vi "setting page 2.vi"() -> (15 "This VI":refnum<vi>)   [LabVIEW 2019]
uses:
  database.lvlib
panel:
  in  "counting device":enum16{"Sensors", "Line Speed", "Sensors&Speed"}(ring)
  in  "IP # speed":string="169.254.12.252"
  out "Error out 7":errorcluster
  out "Error out 6":errorcluster
  out "Error out 5":errorcluster
  out "Error out 4":errorcluster
  out "Error out 3":errorcluster
  out "Error out 2":errorcluster
  out "Error out":errorcluster
  in  "Close Square":bool
  in  "madule path":path=path "C:/Users/DPIS/Desktop/dpis2022/Pallet-car-master/Pallet-car-master/main_func.py"
  in  "high level read thr 3":dbl=25000.0
  in  "high level read thr 2":dbl=25000.0
  in  "box ratio":dbl=8.0
  out "error constant 2":errorcluster
  in  "DB days to save":i16=3
  in  "Debounce Time (s)":dbl=1.0
  in  "counting role 2":T1(ring) caption="counting role"
  in  "ch sw sensor1":dbl
  out "Side Wall Setting":string
  in  "Port":u16=502
  in  "SWL thr":dbl=5000.0
  in  "high level read thr 1":dbl=25000.0
  in  "rising level thr":dbl=50.0
  in  "Database Name":string="dsgs"
  in  "plt number dis":i16=45
  in  "Table Name":string="dpis"
  out "General Setting":string
  in  "SW timout(s)":dbl=1.0
  in  "Curv thr (mm)":dbl=13.0
  in  "SWR thr":dbl=5000.0
  in  "ch sw sensor2":dbl=1.0
  in  "ch sensor3":dbl=6.0
  in  "ch sensor2":dbl=4.0
  in  "ch sensor1":dbl=2.0
  in  "falling Thr sensor 3":dbl=20000.0
  out "Gratebar Setting":string
  in  "max area (hole)":dbl=6000.0
  in  "min area (hole)":dbl=2000.0
  in  "max area size (gap)":dbl=2000.0
  in  "min area size(gap)":dbl=550.0
  in  "max box size":dbl=300000.0
  in  "min box size":dbl=100000.0
  in  "IP #":string="169.254.50.68"
  out "Curve Setting":string
  in  "Img Path":path=path "C:/Users/DPIS/Pictures/pallet pics"
  in  "level2 thr %":u16=50
  in  "level1 thr %":u16=26
  in  "time out":u16=50
  in  "falling Thr sensor 2":dbl=20000.0
  in  "falling Thr sensor 1":dbl=20000.0
  # "DPIS"
  # "SETTING"
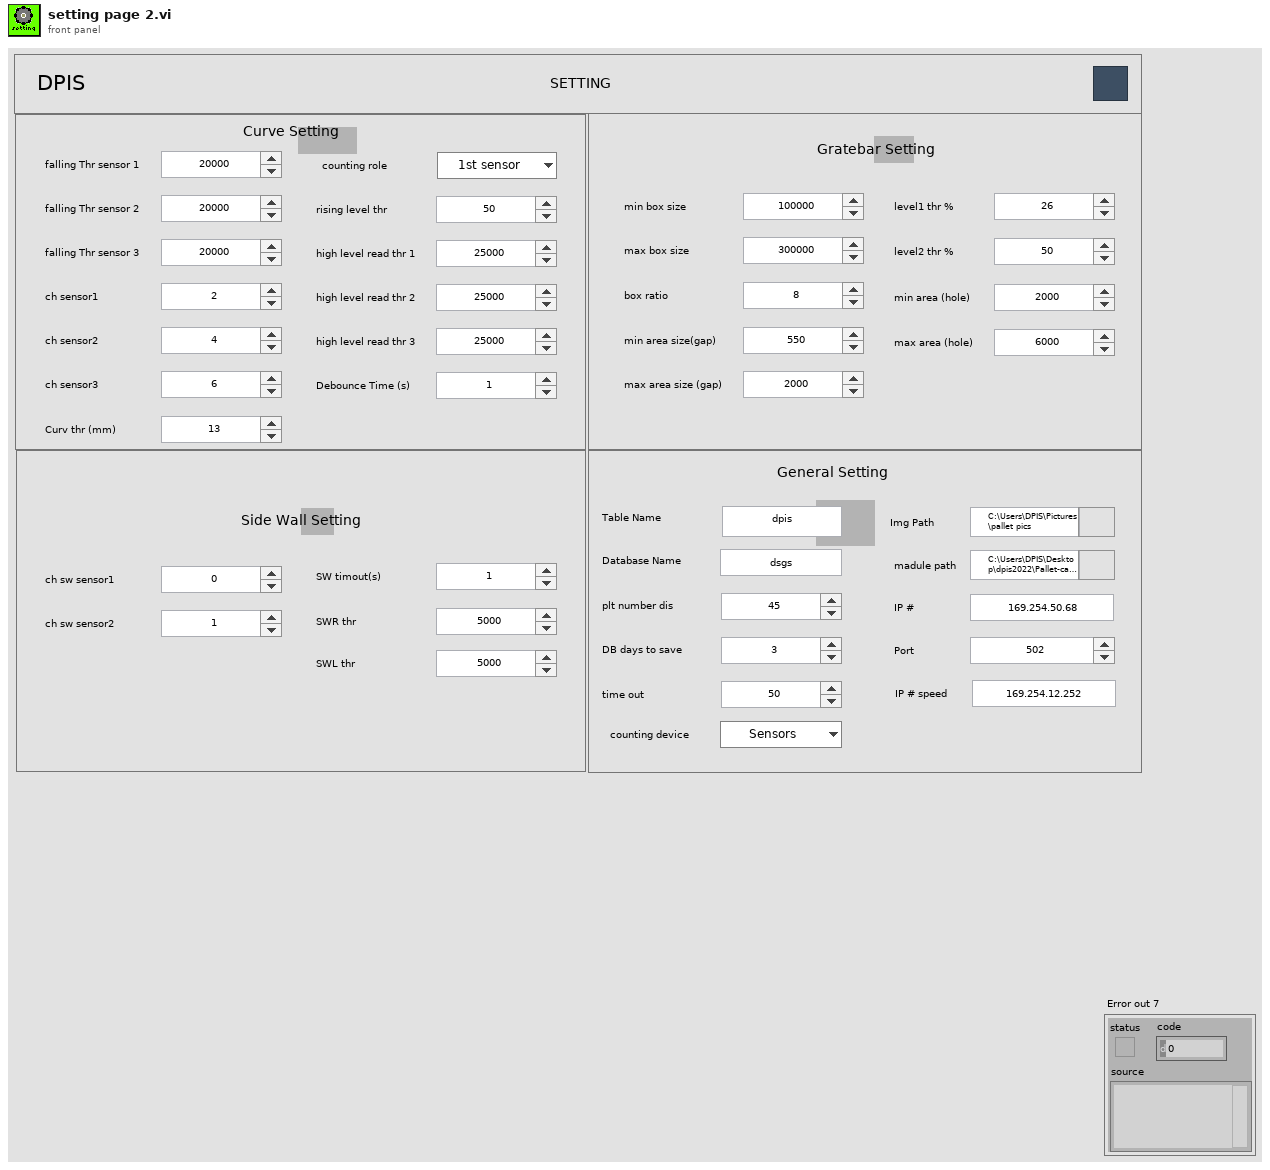
[diagram p1: front panel]
types:
  T1 = enum16{"1st sensor", "2nd sensor", "3rd sensor", "1st+2nd", "1st+3rd", "2nd+3rd", "1st+2nd+3rd"}
  T2 = cluster{i32, string, string, i32, string, path, i32, i32, path, string, "Value":enum16{"Sensors", "Line Speed", "Sensors&Speed"}}
  T3 = cluster{"min box size":dbl, "max box size":dbl, "box ratio":dbl, "min area size(gap)":dbl, "max area size (gap)":dbl, "min area (hole)":dbl, "max area (hole)":dbl}
  T4 = cluster{"ch sensor1":dbl, "ch sensor2":dbl, "chs ensor3":dbl, "ch sw sensor1":dbl, "ch sw sensor2":dbl}
  T5 = cluster{"plt number dis":i16, "Table Name":string, "Database Name":string, "DB days to save":i16, "IP #":string, "Img Path":path, "Port":u16, "time out":u16, "madule path":path}
  T6 = cluster{"high level read thr 1":dbl, "high level read thr 2":dbl, "high level read thr 3":dbl, "Debounce Time (s)":dbl, "rising level thr":dbl, "counting role 2":enum16{"1st sensor", "2nd sensor", "3rd sensor", "1st+2nd", "1st+3rd", "2nd+3rd", "1st+2nd+3rd"}}
  T7 = cluster{"Curv thr (mm)":dbl, "SW timout(s)":dbl, "SWR thr":dbl, "SWL thr ":dbl}
  T8 = cluster{"plt number dis":i16, "Table Name":string, "Database Name":string, "DB days to save":i16, "IP #":string, "Img Path":path, "Port":u16, "time out":u16, "madule path":path, "IP # speed":string, "counting device":enum16{"Sensors", "Line Speed", "Sensors&Speed"}}
  T9 = cluster{"falling Thr sensor 1":dbl, "falling Thr sensor 2":dbl, "falling Thr sensor 3":dbl}
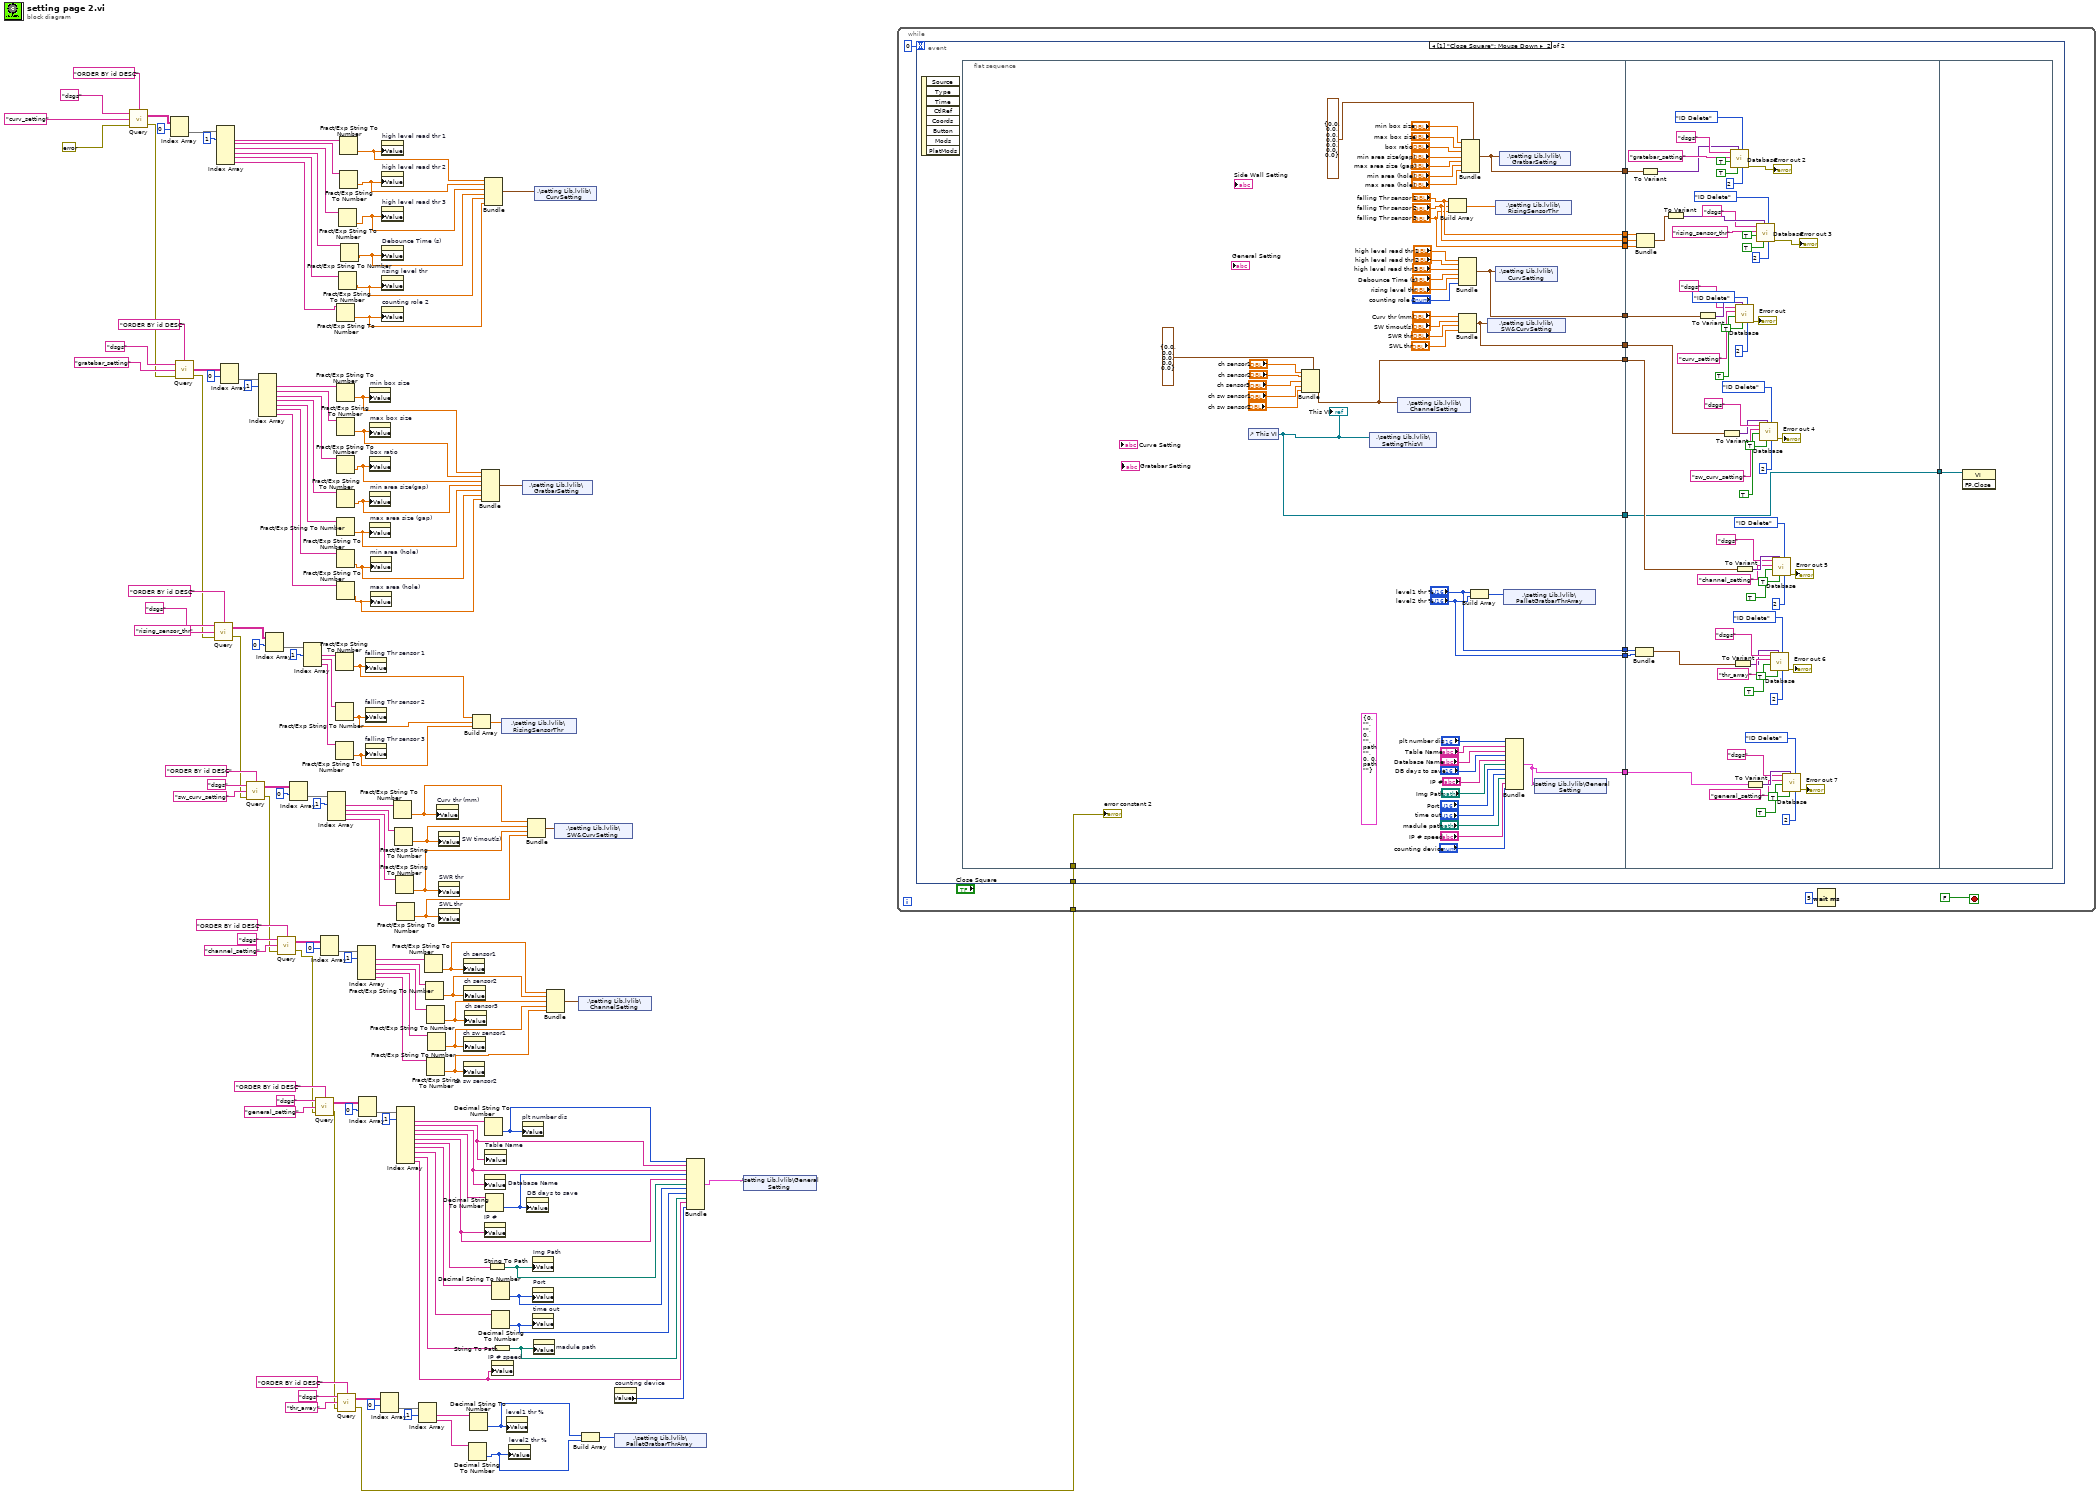
[diagram p0: block diagram]
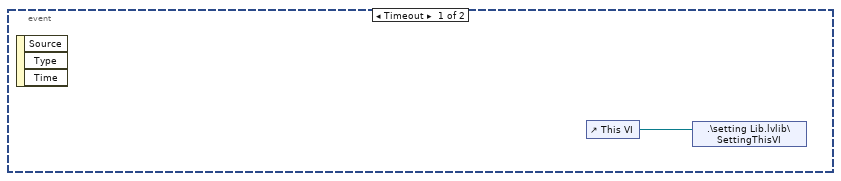
[diagram p2: hidden frame]
diagram:
  n1 = call "Query.vi"("Condition"="ORDER BY id DESC", "Error in"=errorcluster {"status"=FALSE, "code"=0, "source"=""}, "Table Name"="curv_setting", "Connection Name"="dsgs") -> ("Error out"=w106:errorcluster, "data"=w129:string[][])
  n2 = Index Array(array=w129, index (row)=0) -> (element=w131:string[])  [unwired: 1 in]
  n3 = call "Query.vi"("Condition"="ORDER BY id DESC", "Error in"=w106, "Table Name"="gratebar_setting", "Connection Name"="dsgs") -> ("Error out"=w83:errorcluster, "data"=w112:string[][])
  n4 = call "Query.vi"("Condition"="ORDER BY id DESC", "Error in"=w83, "Table Name"="rising_sensor_thr", "Connection Name"="dsgs") -> ("Error out"=w68:errorcluster, "data"=w85:string[][])
  n5 = Index Array(array=w131, index #1=1 ("index")) -> (element #1=w125:string, element #2=w124:string, element #3=w123:string, element #4=w126:string, element #5=w122:string, element #6=w121:string)  [unwired: 5 in]
  n6 = Index Array(array=w112, index (row)=0) -> (element=w110:string[])  [unwired: 1 in]
  n7 = call "Query.vi"("Condition"="ORDER BY id DESC", "Error in"=w68, "Table Name"="sw_curv_setting", "Connection Name"="dsgs") -> ("Error out"=w47:errorcluster, "data"=w74:string[][])
  n8 = Index Array(array=w110, index #1=1 ("index")) -> (element #1=w105:string, element #2=w104:string, element #3=w103:string, element #4=w102:string, element #5=w101:string, element #6=w100:string, element #7=w99:string)  [unwired: 6 in]
  n9 = Index Array(array=w85, index (row)=0) -> (element=w87:string[])  [unwired: 1 in]
  n10 = call "Query.vi"("Condition"="ORDER BY id DESC", "Error in"=w47, "Table Name"="channel_setting", "Connection Name"="dsgs") -> ("Error out"=w32:errorcluster, "data"=w49:string[][])
  n11 = Index Array(array=w74, index (row)=0) -> (element=w72:string[])  [unwired: 1 in]
  n12 = Index Array(array=w87, index #1=1 ("index")) -> (element #1=w82:string, element #2=w81:string, element #3=w80:string)  [unwired: 2 in]
  n13 = call "Query.vi"("Condition"="ORDER BY id DESC", "Error in"=w32, "Table Name"="general_setting", "Connection Name"="dsgs") -> ("Error out"=w9:errorcluster, "data"=w38:string[][])
  n14 = Index Array(array=w49, index (row)=0) -> (element=w51:string[])  [unwired: 1 in]
  n15 = Index Array(array=w72, index #1=1 ("index")) -> (element #1=w67:string, element #2=w66:string, element #3=w65:string, element #4=w64:string)  [unwired: 3 in]
  n16 = Fract/Exp String To Number(string=w82) -> (number=w79:dbl)  [unwired: 3 in, 1 out]
  n17 = Fract/Exp String To Number(string=w81) -> (number=w78:dbl)  [unwired: 3 in, 1 out]
  n18 = Fract/Exp String To Number(string=w80) -> (number=w77:dbl)  [unwired: 3 in, 1 out]
  n19 = Fract/Exp String To Number(string=w105) -> (number=w98:dbl)  [unwired: 3 in, 1 out]
  n20 = Fract/Exp String To Number(string=w104) -> (number=w97:dbl)  [unwired: 3 in, 1 out]
  n21 = Fract/Exp String To Number(string=w103) -> (number=w96:dbl)  [unwired: 3 in, 1 out]
  n22 = Fract/Exp String To Number(string=w102) -> (number=w95:dbl)  [unwired: 3 in, 1 out]
  n23 = Fract/Exp String To Number(string=w101) -> (number=w94:dbl)  [unwired: 3 in, 1 out]
  n24 = Fract/Exp String To Number(string=w121) -> (number=w115:dbl)  [unwired: 3 in, 1 out]
  n25 = Fract/Exp String To Number(string=w100) -> (number=w93:dbl)  [unwired: 3 in, 1 out]
  n26 = Fract/Exp String To Number(string=w99) -> (number=w92:dbl)  [unwired: 3 in, 1 out]
  n27 = call "Query.vi"("Condition"="ORDER BY id DESC", "Error in"=w9, "Table Name"="thr_array", "Connection Name"="dsgs") -> ("Error out"=w135:errorcluster, "data"=w11:string[][])
  n28 = Fract/Exp String To Number(string=w122) -> (number=w116:dbl)  [unwired: 3 in, 1 out]
  n29 = Fract/Exp String To Number(string=w123) -> (number=w118:dbl)  [unwired: 3 in, 1 out]
  n30 = Fract/Exp String To Number(string=w125) -> (number=w120:dbl)  [unwired: 3 in, 1 out]
  n31 = Fract/Exp String To Number(string=w124) -> (number=w119:dbl)  [unwired: 3 in, 1 out]
  n32 = Fract/Exp String To Number(string=w126) -> (number=w117:dbl)  [unwired: 3 in, 1 out]
  n33 = Index Array(array=w51, index #1=1 ("index")) -> (element #1=w55:string, element #2=w56:string, element #3=w57:string, element #4=w58:string, element #5=w46:string)  [unwired: 4 in]
  n34 = Index Array(array=w38, index (row)=0) -> (element=w36:string[])  [unwired: 1 in]
  n35 = property on="falling Thr sensor 1" class="DigNum (strict)"("Value"=w79) -> ()  [unwired: 2 in, 2 out]
  n36 = property on="falling Thr sensor 2" class="DigNum (strict)"("Value"=w78) -> ()  [unwired: 2 in, 2 out]
  n37 = property on="falling Thr sensor 3" class="DigNum (strict)"("Value"=w77) -> ()  [unwired: 2 in, 2 out]
  n38 = property on="min box size" class="DigNum (strict)"("Value"=w98) -> ()  [unwired: 2 in, 2 out]
  n39 = property on="max box size" class="DigNum (strict)"("Value"=w97) -> ()  [unwired: 2 in, 2 out]
  n40 = property on="box ratio" class="DigNum (strict)"("Value"=w96) -> ()  [unwired: 2 in, 2 out]
  n41 = property on="min area size(gap)" class="DigNum (strict)"("Value"=w95) -> ()  [unwired: 2 in, 2 out]
  n42 = property on="max area size (gap)" class="DigNum (strict)"("Value"=w94) -> ()  [unwired: 2 in, 2 out]
  n43 = property on="min area (hole)" class="DigNum (strict)"("Value"=w93) -> ()  [unwired: 2 in, 2 out]
  n44 = property on="max area (hole)" class="DigNum (strict)"("Value"=w92) -> ()  [unwired: 2 in, 2 out]
  n45 = Index Array(array=w11, index (row)=0) -> (element=w13:string[])  [unwired: 1 in]
  n46 = property on="high level read thr 1" class="DigNum (strict)"("Value"=w120) -> ()  [unwired: 2 in, 2 out]
  n47 = property on="high level read thr 2" class="DigNum (strict)"("Value"=w119) -> ()  [unwired: 2 in, 2 out]
  n48 = property on="high level read thr 3" class="DigNum (strict)"("Value"=w118) -> ()  [unwired: 2 in, 2 out]
  n49 = property on="Debounce Time (s)" class="DigNum (strict)"("Value"=w117) -> ()  [unwired: 2 in, 2 out]
  n50 = property on="rising level thr" class="DigNum (strict)"("Value"=w116) -> ()  [unwired: 2 in, 2 out]
  n51 = property on="counting role 2" class="Enum (strict)"("Value"=w115) -> ()  [unwired: 2 in, 2 out]
  n52 = Fract/Exp String To Number(string=w67) -> (number=w63:dbl)  [unwired: 3 in, 1 out]
  n53 = Fract/Exp String To Number(string=w66) -> (number=w62:dbl)  [unwired: 3 in, 1 out]
  n54 = Fract/Exp String To Number(string=w65) -> (number=w61:dbl)  [unwired: 3 in, 1 out]
  n55 = Index Array(array=w36, index #1=1 ("index")) -> (element #1=w31:string, element #2=w25:string, element #3=w24:string, element #4=w23:string, element #5=w22:string, element #6=w30:string, element #7=w29:string, element #8=w28:string, element #9=w27:string, element #10=w3:string)  [unwired: 9 in]
  n56 = Fract/Exp String To Number(string=w64) -> (number=w60:dbl)  [unwired: 3 in, 1 out]
  n57 = Index Array(array=w13, index #1=1 ("index")) -> (element #1=w8:string, element #2=w7:string)  [unwired: 1 in]
  n58 = Fract/Exp String To Number(string=w55) -> (number=w45:dbl)  [unwired: 3 in, 1 out]
  n59 = Fract/Exp String To Number(string=w56) -> (number=w44:dbl)  [unwired: 3 in, 1 out]
  n60 = Fract/Exp String To Number(string=w57) -> (number=w43:dbl)  [unwired: 3 in, 1 out]
  n61 = Fract/Exp String To Number(string=w46) -> (number=w41:dbl)  [unwired: 3 in, 1 out]
  n62 = Fract/Exp String To Number(string=w58) -> (number=w42:dbl)  [unwired: 3 in, 1 out]
  n63 = property on="Curv thr (mm)" class="DigNum (strict)"("Value"=w63) -> ()  [unwired: 2 in, 2 out]
  n64 = property on="SW timout(s)" class="DigNum (strict)"("Value"=w62) -> ()  [unwired: 2 in, 2 out]
  n65 = property on="SWR thr" class="DigNum (strict)"("Value"=w61) -> ()  [unwired: 2 in, 2 out]
  n66 = property on="SWL thr" class="DigNum (strict)"("Value"=w60) -> ()  [unwired: 2 in, 2 out]
  n67 = property on="ch sensor1" class="DigNum (strict)"("Value"=w45) -> ()  [unwired: 2 in, 2 out]
  n68 = property on="ch sw sensor2" class="DigNum (strict)"("Value"=w41) -> ()  [unwired: 2 in, 2 out]
  n69 = property on="ch sensor2" class="DigNum (strict)"("Value"=w44) -> ()  [unwired: 2 in, 2 out]
  n70 = property on="ch sw sensor1" class="DigNum (strict)"("Value"=w42) -> ()  [unwired: 2 in, 2 out]
  n71 = property on="ch sensor3" class="DigNum (strict)"("Value"=w43) -> ()  [unwired: 2 in, 2 out]
  n72 = Decimal String To Number(string=w7) -> (number=w4:i32)  [unwired: 2 in, 1 out]
  n73 = Decimal String To Number(string=w8) -> (number=w5:i32)  [unwired: 2 in, 1 out]
  n74 = Build Array(w79, w78, w77) -> (w76:dbl[])
  n75 = Bundle(w98, w97, w96, w95, w94, w93, w92) -> (w91:cluster{dbl, dbl, dbl, dbl, dbl, dbl, dbl})  [unwired: 1 in]
  n76 = Decimal String To Number(string=w31) -> (number=w26:i32)  [unwired: 2 in, 1 out]
  n77 = property on="Database Name" class="Str"("Value"=w24) -> ()  [unwired: 2 in, 2 out]
  n78 = property on="IP #" class="Str"("Value"=w22) -> ()  [unwired: 2 in, 2 out]
  n79 = Bundle(w120, w119, w118, w117, w116, w115) -> (w114:cluster{dbl, dbl, dbl, dbl, dbl, dbl})  [unwired: 1 in]
  n80 = property on="Table Name" class="Str"("Value"=w25) -> ()  [unwired: 2 in, 2 out]
  n81 = Decimal String To Number(string=w23) -> (number=w21:i32)  [unwired: 2 in, 1 out]
  n82 = String To Path(string=w30) -> (path=w20:path)
  n83 = Decimal String To Number(string=w29) -> (number=w19:i32)  [unwired: 2 in, 1 out]
  n84 = Decimal String To Number(string=w28) -> (number=w18:i32)  [unwired: 2 in, 1 out]
  n85 = property on="IP # speed" class="Str"("Value"=w3) -> ()  [unwired: 2 in, 2 out]
  n86 = String To Path(string=w27) -> (path=w17:path)
  n87 = shared-variable ".\\setting Lib.lvlib\\RisingSensorThr"(w76) -> ()  [unwired: 1 in, 1 out]
  n88 = property on="level1 thr %" class="DigNum (strict)"("Value"=w5) -> ()  [unwired: 2 in, 2 out]
  n89 = property on="level2 thr %" class="DigNum (strict)"("Value"=w4) -> ()  [unwired: 2 in, 2 out]
  n90 = shared-variable ".\\setting Lib.lvlib\\GratbarSetting"(w91) -> ()  [unwired: 1 in, 1 out]
  n91 = property on="plt number dis" class="DigNum (strict)"("Value"=w26) -> ()  [unwired: 2 in, 2 out]
  n92 = property on="DB days to save" class="DigNum (strict)"("Value"=w21) -> ()  [unwired: 2 in, 2 out]
  n93 = Bundle(w63, w62, w61, w60) -> (w59:cluster{dbl, dbl, dbl, dbl})  [unwired: 1 in]
  n94 = property on="Img Path" class="Path"("Value"=w20) -> ()  [unwired: 2 in, 2 out]
  n95 = property on="Port" class="DigNum (strict)"("Value"=w19) -> ()  [unwired: 2 in, 2 out]
  n96 = property on="time out" class="DigNum (strict)"("Value"=w18) -> ()  [unwired: 2 in, 2 out]
  n97 = property on="madule path" class="Path"("Value"=w17) -> ()  [unwired: 2 in, 2 out]
  n98 = shared-variable ".\\setting Lib.lvlib\\CurvSetting"(w114) -> ()  [unwired: 1 in, 1 out]
  n99 = Bundle(w45, w44, w43, w42, w41) -> (w40:cluster{dbl, dbl, dbl, dbl, dbl})  [unwired: 1 in]
  n100 = shared-variable ".\\setting Lib.lvlib\\SW&CurvSetting"(w59) -> ()  [unwired: 1 in, 1 out]
  n101 = shared-variable ".\\setting Lib.lvlib\\ChannelSetting"(w40) -> ()  [unwired: 1 in, 1 out]
  n102 = Build Array(w5, w4) -> (w6:i32[])
  n103 = shared-variable ".\\setting Lib.lvlib\\PalletGratbarThrArray"(w6) -> ()  [unwired: 1 in, 1 out]
  n104 = property on="counting device" class="Enum (strict)"() -> ("Value"=w1:enum16{"Sensors", "Line Speed", "Sensors&Speed"})  [unwired: 2 in, 2 out]
  n105 = Bundle(w26, w25, w24, w21, w22, w20, w19, w18, w17, w3, "Value"=w1) -> (w2:T2)  [unwired: 1 in]
  n106 = shared-variable ".\\setting Lib.lvlib\\General Setting"(w2) -> ()  [unwired: 1 in, 1 out]
  n107 = while {
    tunnel: w135 -> [w138]
    stop <- FALSE stop-if-true
    n108 = event shown="[1] \"Close Square\": Mouse Down" {
      selector: _ -> [_ _]
      dyn-events: _ -> [_ _]
      timeout: 0 -> [_ _]
      tunnel: w138 -> [_ w143]
      event Timeout {
        n109 = event-data() -> ()  [unwired: 1 in, 3 out]
        n110 = control-ref of="This VI"() -> (w140:refnum<vi>)
        n111 = shared-variable ".\\setting Lib.lvlib\\SettingThisVI"(w140) -> ()  [unwired: 1 in, 1 out]
      }
      event "Close Square": Mouse Down {
        n112 = event-data() -> ()  [unwired: 1 in, 8 out]
        n113 = flat-sequence {
          tunnel: ["falling Thr sensor 1"] -> w153
          tunnel: ["falling Thr sensor 2"] -> w152
          tunnel: ["falling Thr sensor 3"] -> w151
          tunnel: [w165] -> w150
          tunnel: [w164] -> w149
          tunnel: [w163] -> w148
          tunnel: [w161] -> w147
          tunnel: ["level1 thr %"] -> w146
          tunnel: ["level2 thr %"] -> w145
          tunnel: [w154] -> w144
          tunnel: w143 -> [w158]
          tunnel: [w157] -> w141
          tunnel: w153 -> [w248]
          tunnel: w152 -> [w247]
          tunnel: w151 -> [w246]
          tunnel: w150 -> [w224]
          tunnel: w149 -> [w258]
          tunnel: w148 -> [w262]
          tunnel: w147 -> [w237]
          tunnel: w146 -> [w215]
          tunnel: w145 -> [w214]
          tunnel: w144 -> [w204]
          tunnel: [w203] -> w142
          tunnel: w141 -> [w203]
          tunnel: w142 -> [w272]
          frame #0 {
            (unwired) T5 {"plt number dis"=0, "Table Name"="", "Database Name"="", "DB days to save"=0, "IP #"="", "Img Path"=path "", "Port"=0, "time out"=0, "madule path"=path ""} ("cluster")
            n114 = control-ref of="This VI"() -> (w157:refnum<vi>)
            "This VI" <- w157
            n115 = Bundle(cluster=T4 {"ch sensor1"=0.0, "ch sensor2"=0.0, "chs ensor3"=0.0, "ch sw sensor1"=0.0, "ch sw sensor2"=0.0}, "ch sensor1"="ch sensor1", "ch sensor2"="ch sensor2", "chs ensor3"="ch sensor3", "ch sw sensor1"="ch sw sensor1", "ch sw sensor2"="ch sw sensor2") -> (w165:T4)
            n116 = shared-variable ".\\setting Lib.lvlib\\SettingThisVI"(w157) -> ()  [unwired: 1 in, 1 out]
            n117 = shared-variable ".\\setting Lib.lvlib\\ChannelSetting"(w165) -> ()  [unwired: 1 in, 1 out]
            n118 = Build Array("falling Thr sensor 1", "falling Thr sensor 2", "falling Thr sensor 3") -> (w162:dbl[])
            n119 = Bundle("high level read thr 1"="high level read thr 1", "high level read thr 2"="high level read thr 2", "high level read thr 3"="high level read thr 3", "Debounce Time (s)"="Debounce Time (s)", "rising level thr"="rising level thr", "counting role 2"="counting role 2") -> (w164:T6)  [unwired: 1 in]
            n120 = Bundle("Curv thr (mm)"="Curv thr (mm)", "SW timout(s)"="SW timout(s)", "SWR thr"="SWR thr", "SWL thr"="SWL thr") -> (w161:T7)  [unwired: 1 in]
            n121 = Bundle(cluster=T3 {"min box size"=0.0, "max box size"=0.0, "box ratio"=0.0, "min area size(gap)"=0.0, "max area size (gap)"=0.0, "min area (hole)"=0.0, "max area (hole)"=0.0}, "min box size"="min box size", "max box size"="max box size", "box ratio"="box ratio", "min area size(gap)"="min area size(gap)", "max area size (gap)"="max area size (gap)", "min area (hole)"="min area (hole)", "max area (hole)"="max area (hole)") -> (w163:T3)
            n122 = Build Array("level1 thr %", "level2 thr %") -> (w187:u16[])
            n123 = shared-variable ".\\setting Lib.lvlib\\SW&CurvSetting"(w161) -> ()  [unwired: 1 in, 1 out]
            n124 = shared-variable ".\\setting Lib.lvlib\\RisingSensorThr"(w162) -> ()  [unwired: 1 in, 1 out]
            n125 = shared-variable ".\\setting Lib.lvlib\\CurvSetting"(w164) -> ()  [unwired: 1 in, 1 out]
            n126 = shared-variable ".\\setting Lib.lvlib\\GratbarSetting"(w163) -> ()  [unwired: 1 in, 1 out]
            n127 = shared-variable ".\\setting Lib.lvlib\\PalletGratbarThrArray"(w187) -> ()  [unwired: 1 in, 1 out]
            n128 = Bundle("plt number dis"="plt number dis", "Table Name"="Table Name", "Database Name"="Database Name", "DB days to save"="DB days to save", "IP #"="IP #", "Img Path"="Img Path", "Port"="Port", "time out"="time out", "madule path"="madule path", "IP # speed"="IP # speed", "counting device"="counting device") -> (w154:T8)  [unwired: 1 in]
            n129 = shared-variable ".\\setting Lib.lvlib\\General Setting"(w154) -> ()  [unwired: 1 in, 1 out]
            "error constant 2" <- w158
          }
          frame #1 {
            n130 = Bundle("level1 thr %"=w215, "level2 thr %"=w214) -> (w213:cluster{"level1 thr %":u16, "level2 thr %":u16})  [unwired: 1 in]
            n131 = Bundle("falling Thr sensor 1"=w248, "falling Thr sensor 2"=w247, "falling Thr sensor 3"=w246) -> (w245:T9)  [unwired: 1 in]
            n132 = To Variant(anything=w262) -> (Variant=w261:variant)
            n133 = To Variant(anything=w245) -> (Variant=w251:variant)
            n134 = To Variant(anything=w258) -> (Variant=w271:variant)
            n135 = To Variant(anything=w237) -> (Variant=w238:variant)
            n136 = call "Database.vi"("Maximum Row"=2, "Enum"=enum16{"ID Delete", "Time Delete"}."ID Delete", "Delete row?"=TRUE, "Data"=w261, "Auto Increment ID?"=TRUE, "Table"="gratebar_setting", "Connection"="dsgs") -> ("Error out"=→"Error out 2":errorcluster)  [unwired: 4 in]
            n137 = To Variant(anything=w213) -> (Variant=w217:variant)
            n138 = call "Database.vi"("Maximum Row"=2, "Enum"=enum16{"ID Delete", "Time Delete"}."ID Delete", "Delete row?"=TRUE, "Data"=w271, "Auto Increment ID?"=TRUE, "Table"="curv_setting", "Connection"="dsgs") -> ("Error out"=→"Error out":errorcluster)  [unwired: 4 in]
            n139 = To Variant(anything=w224) -> (Variant=w231:variant)
            n140 = To Variant(anything=w204) -> (Variant=w211:variant)
            n141 = call "Database.vi"("Maximum Row"=2, "Enum"=enum16{"ID Delete", "Time Delete"}."ID Delete", "Delete row?"=TRUE, "Data"=w251, "Auto Increment ID?"=TRUE, "Table"="rising_sensor_thr", "Connection"="dsgs") -> ("Error out"=→"Error out 3":errorcluster)  [unwired: 4 in]
            n142 = call "Database.vi"("Maximum Row"=2, "Enum"=enum16{"ID Delete", "Time Delete"}."ID Delete", "Delete row?"=TRUE, "Data"=w238, "Auto Increment ID?"=TRUE, "Table"="sw_curv_setting", "Connection"="dsgs") -> ("Error out"=→"Error out 4":errorcluster)  [unwired: 4 in]
            n143 = call "Database.vi"("Maximum Row"=2, "Enum"=enum16{"ID Delete", "Time Delete"}."ID Delete", "Delete row?"=TRUE, "Data"=w217, "Auto Increment ID?"=TRUE, "Table"="thr_array", "Connection"="dsgs") -> ("Error out"=→"Error out 6":errorcluster)  [unwired: 4 in]
            n144 = call "Database.vi"("Maximum Row"=2, "Enum"=enum16{"ID Delete", "Time Delete"}."ID Delete", "Delete row?"=TRUE, "Data"=w231, "Auto Increment ID?"=TRUE, "Table"="channel_setting", "Connection"="dsgs") -> ("Error out"=→"Error out 5":errorcluster)  [unwired: 4 in]
            n145 = call "Database.vi"("Maximum Row"=2, "Enum"=enum16{"ID Delete", "Time Delete"}."ID Delete", "Delete row?"=TRUE, "Data"=w211, "Auto Increment ID?"=TRUE, "Table"="general_setting", "Connection"="dsgs") -> ("Error out"=→"Error out 7":errorcluster)  [unwired: 4 in]
          }
          frame #2 {
            n146 = invoke class="VI" method="FP.Close"(reference=w272) -> ()  [unwired: 2 in, 3 out]
          }
        }
      }
    }
    n147 = Wait (ms)(milliseconds to wait=u32 5) -> ()  [unwired: 1 out]
  }
